vi "Copy_Proj_Data.vi"(8 "error in (no error)":errorcluster, 9 "IB_Destination.lvclass":refnum<class "IB_Destination.lvclass">, 10 "IB_Tree_Item_Proj in":refnum<class "IB_Tree_Item_Proj.lvclass">, 11 "IB_Source in":refnum<class "IB_Source.lvclass">) -> (0 "error out":errorcluster, 3 "IB_Source out":refnum<class "IB_Source.lvclass">)   [LabVIEW 2020, in "IB_Source.lvclass"]
uses:
  <vilib>/AppBuilder/IB_Classes/Source/IB_Source.lvclass
  <vilib>/AppBuilder/IB_Classes/Source/IB_Source.lvclass/IB_Source.ctl
  <vilib>/AppBuilder/IB_Classes/Tree_Item/IB_Tree_Item.lvclass
  <vilib>/AppBuilder/IB_Classes/Tree_Item_Proj/IB_Tree_Item_Proj.lvclass
  <vilib>/AppBuilder/IB_Classes/Destination/IB_Destination.lvclass
  e:/builds/penguin/labview/branches/2020/dev/dist/vi.lib/AppBuilder/IB_Classes/Tree_Item/IB_Tree_Item.lvclass
  e:/builds/penguin/labview/branches/2020/dev/dist/vi.lib/AppBuilder/IB_Classes/Tree_Item_Proj/IB_Tree_Item_Proj.lvclass
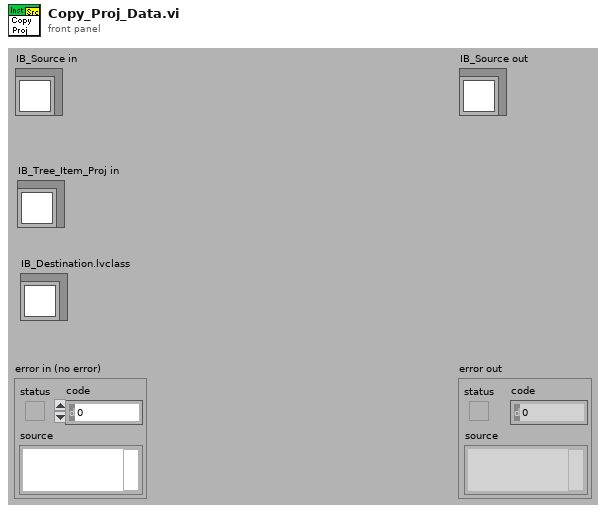
[diagram p1: front panel]
types:
  T1 = typedef "IB_Destination.ctl" = cluster{"name":string, "unlock":bool, "parentTag":string, "destTag":string, "eng_installPath":string}
  T2 = typedef "IB_Tree_Item.ctl" = cluster{"symbol index":i32, "child tag":string, "parentTag":string, "left cell name":string}
  T3 = typedef "IB_Tree_Item_Proj.ctl" = cluster{"itemID":string, "path":path}
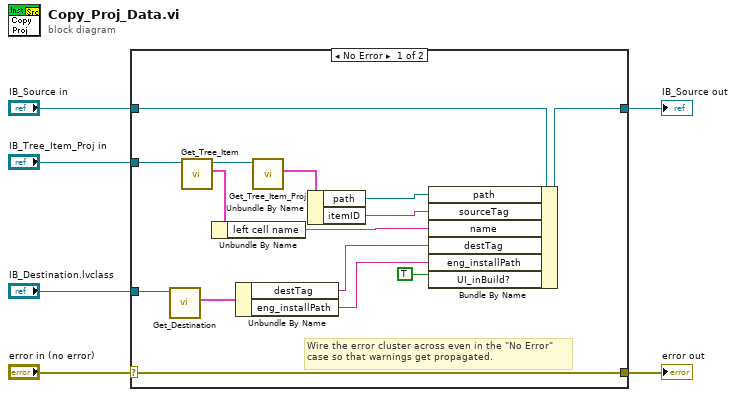
[diagram p0: block diagram]
diagram:
  n1 = case shown="No Error" "error in (no error)" {
    selector: "error in (no error)" -> [w21 w23]
    tunnel: [w21 w23] -> w5
    tunnel: [w13 w22] -> w3
    tunnel: "IB_Source in" -> [w14 w22]
    tunnel: "IB_Tree_Item_Proj in" -> [w12 _]
    tunnel: "IB_Destination.lvclass" -> [w11 _]
    frame No Error {
      # "Wire the error cluster across even in the \"No Error\"\ncase so that warnings get propagated."
      n2 = call <vilib>:"Get_Destination.vi"("IB_Destination in"=w11) -> ("data"=w10:T1)  [unwired: 8 in, 2 out]
      n3 = call <vilib>:"Get_Tree_Item.vi"("IB_TreeItem in"=w12) -> ("data"=w19:T2, "IB_TreeItem out"=w20:refnum<class "IB_Tree_Item_Proj.lvclass">)  [unwired: 8 in, 1 out]
      n4 = Unbundle By Name(w19) -> ("left cell name"=w17:string)
      n5 = Unbundle By Name(w10) -> ("destTag"=w8:string, "eng_installPath"=w9:string)
      n6 = call <vilib>:"Get_Tree_Item_Proj.vi"("IB_TreeProjectItem in"=w20) -> ("data"=w18:T3)  [unwired: 8 in, 2 out]
      n7 = Unbundle By Name(w18) -> ("path"=w15:path, "itemID"=w16:string)
      n8 = Bundle By Name(cluster=w14, "path"=w15, "sourceTag"=w16, "name"=w17, "destTag"=w8, "eng_installPath"=w9, "UI_inBuild?"=TRUE ("data.UI_inBuild?")) -> (w13:refnum<class "IB_Source.lvclass">)
    }
    frame Error {
    }
  }
  "error out" <- w5
  "IB_Source out" <- w3
